vi "Mult Scalar.vi"(8 "error in":errorcluster, 10 "Scale":dbl, 11 "Vec3d in":refnum<class "Vec3d Class.lvclass">) -> (0 "error out":errorcluster, 3 "Vec3d out":refnum<class "Vec3d Class.lvclass">)   [LabVIEW 2011, in "Vec3d Class.lvclass"]
uses:
  Vec3d Class.lvclass
  Vec3d Class.lvclass/Vec3d Class.ctl
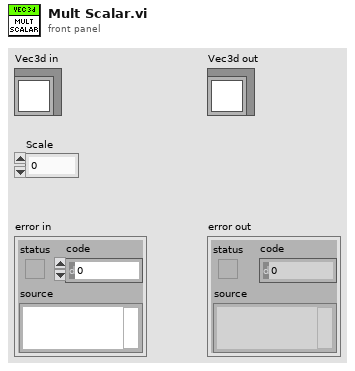
[diagram p1: front panel]
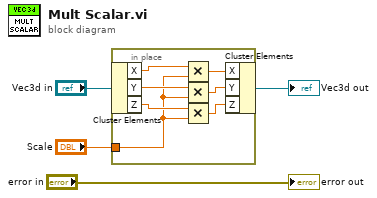
[diagram p0: block diagram]
diagram:
  n1 = in-place {
    in-place-border: "Scale" -> [w8]
    n2 = in-place-cluster #1("Vec3d in") -> ("X"=w10:dbl, "Y"=w11:dbl, "Z"=w9:dbl)
    n3 = Multiply(x=w10, y=w8) -> (x*y=w7:dbl)
    n4 = Multiply(x=w11, y=w8) -> (x*y=w6:dbl)
    n5 = Multiply(x=w9, y=w8) -> (x*y=w5:dbl)
    n6 = in-place-cluster #1("X"=w7, "Y"=w6, "Z"=w5) -> (→"Vec3d out":refnum<class "Vec3d Class.lvclass">)
  }
  "error out" <- "error in"
